vi "_PC_RTLoop_RTSysResource.vi"(7 "Function":enum16{"Init", "Get Data", "Close"}(ring)=enum."Get Data", 8 "error in (no error)":errorcluster, 11 "RT Resource XY Graph":refnum<vi>) -> (0 "error out":errorcluster)   [LabVIEW 2018]
uses:
  <resource>/objmgr/ni.var.rc
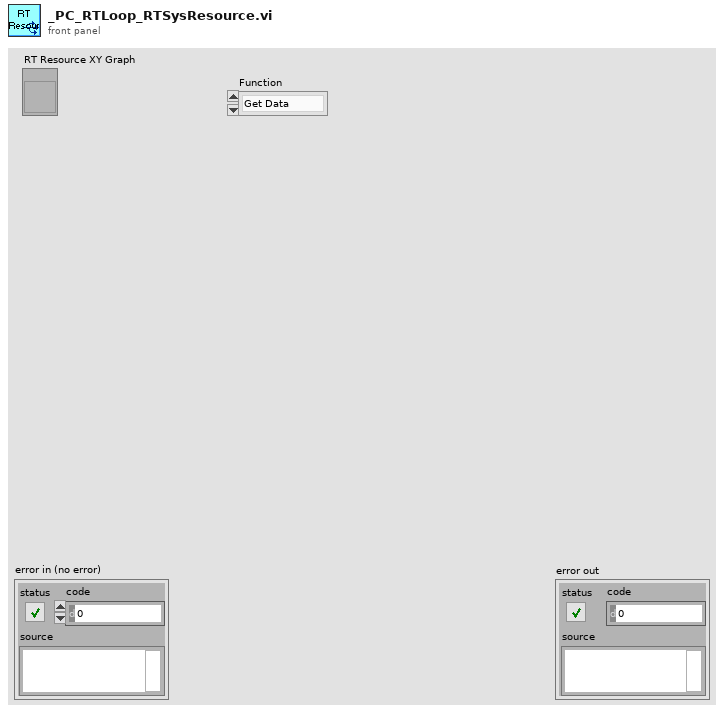
[diagram p1: front panel]
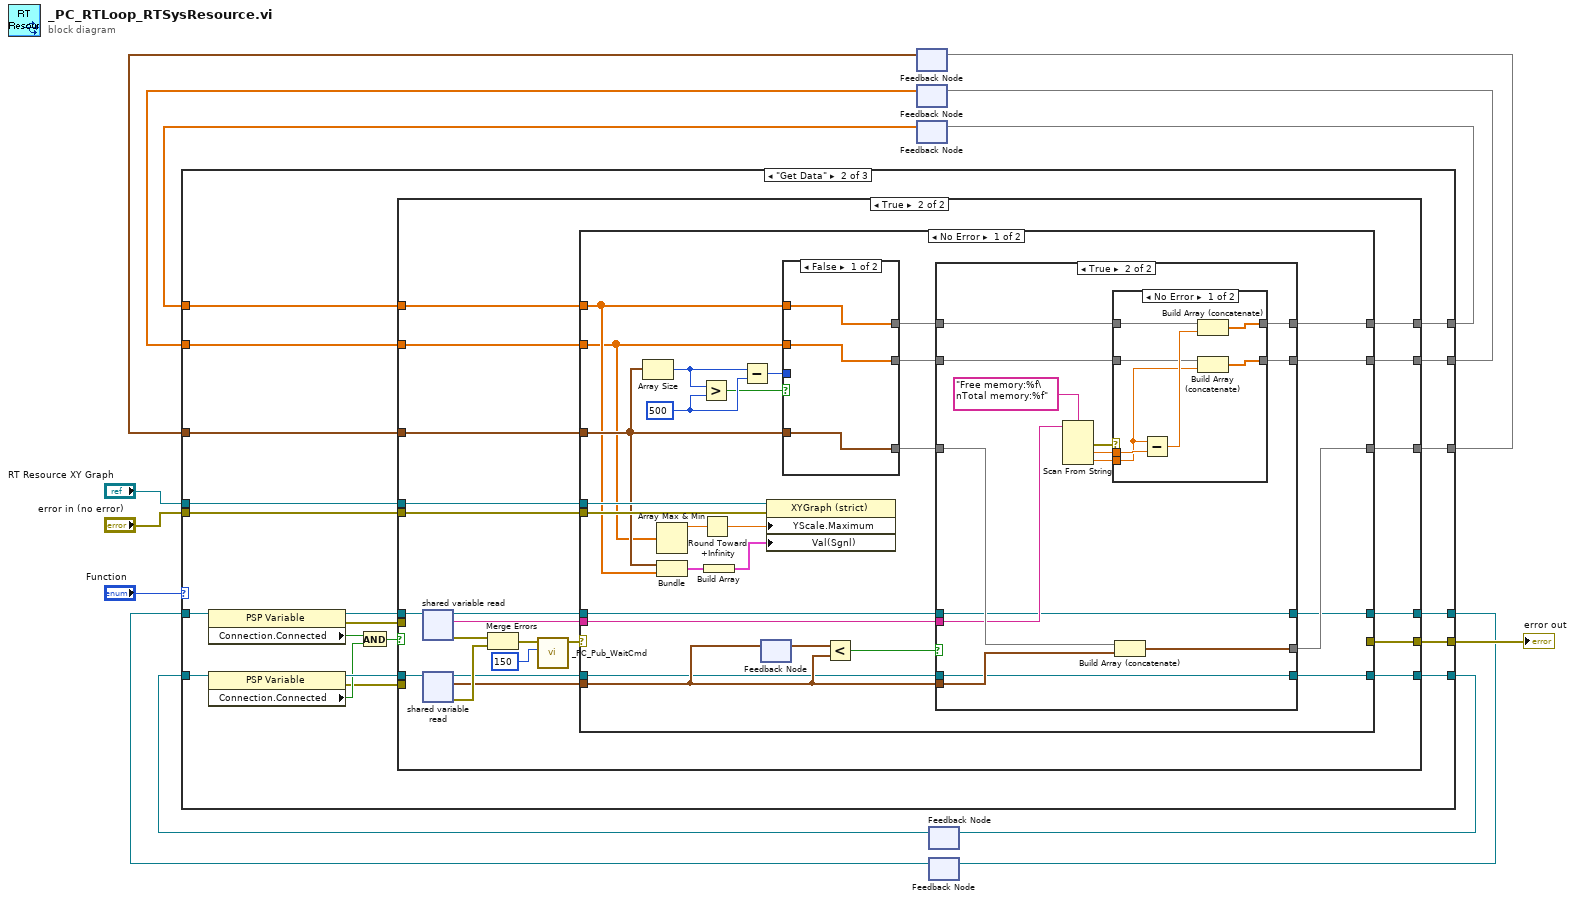
[diagram p0: block diagram]
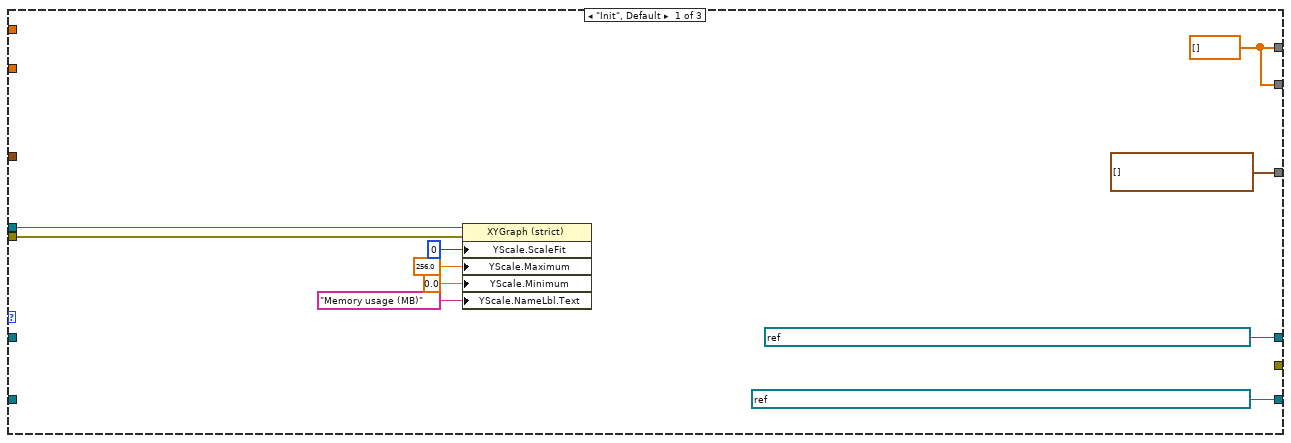
[diagram p2: hidden frame]
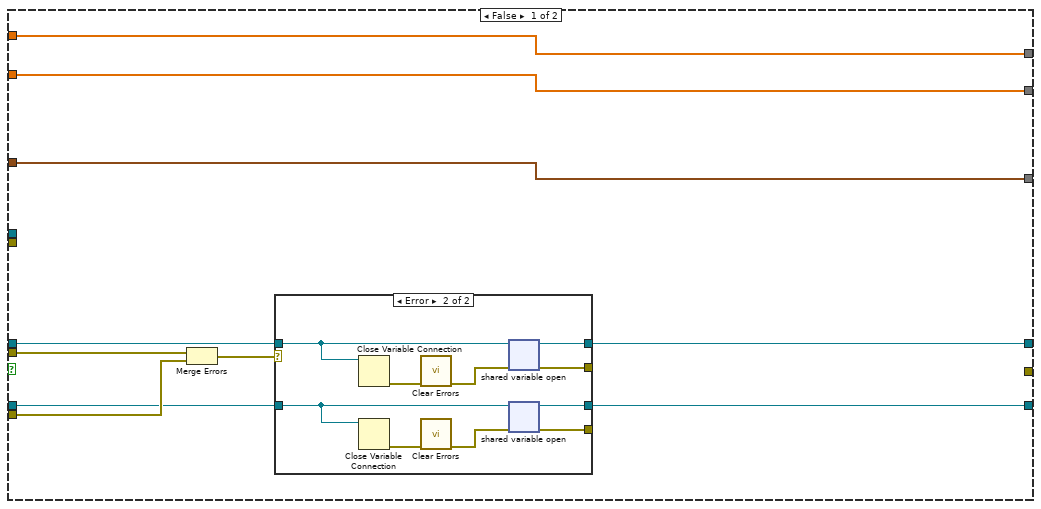
[diagram p3: hidden frame]
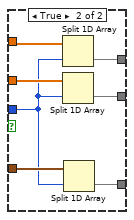
[diagram p7: hidden frame]
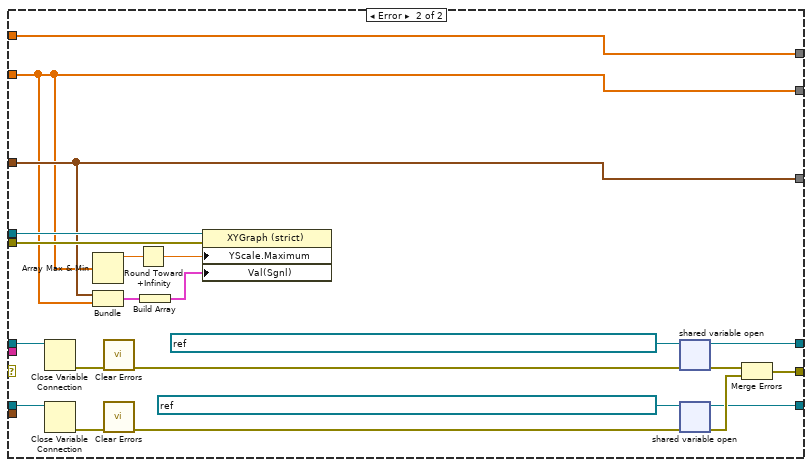
[diagram p8: hidden frame]
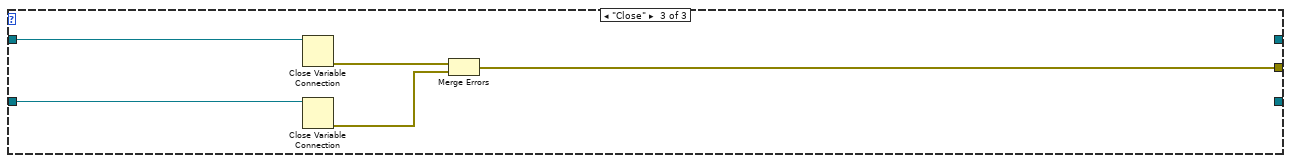
[diagram p9: hidden frame]
diagram:
  n1 = feedback #1() -> (w9:timestamp[])  [unwired: 1 in]
  n2 = feedback #2() -> (w11:dbl[])  [unwired: 1 in]
  n3 = feedback #3() -> (w13:dbl[])  [unwired: 1 in]
  n4 = feedback #4() -> (w5:refnum<k21>)  [unwired: 1 in]
  n5 = feedback #5() -> (w4:refnum<k21>)  [unwired: 1 in]
  n6 = case shown="\"Get Data\"" "Function" {
    tunnel: [w22 w44 _] -> w14
    tunnel: w13 -> [_ w43 _]
    tunnel: [w22 w42 _] -> w12
    tunnel: w11 -> [_ w41 _]
    tunnel: [timestamp[] [] w40 _] -> w10
    tunnel: w9 -> [_ w39 _]
    tunnel: [_ w38 w176] -> w8
    tunnel: [refnum<k21> "ni.var.psp://NI-sbRIO/_RT_CtrlLoop_ResourcesMonitor_Variables/RT_SysTimeStamp" ("shared variable refnum in") w37 _] -> w7
    tunnel: [refnum<k21> "ni.var.psp://NI-sbRIO/_RT_CtrlLoop_ResourcesMonitor_Variables/ResourceUsage" ("shared variable refnum in") w36 _] -> w6
    tunnel: w4 -> [_ w35 w180]
    tunnel: w5 -> [_ w34 w179]
    tunnel: "RT Resource XY Graph" -> [w16 w33 _]
    tunnel: "error in (no error)" -> [w15 w32 _]
    frame "Init", Default {
      w22 = dbl[] []
      n7 = property class="XYGraph (strict)"(reference=w16, error in=w15, "YScale.ScaleFit"=u8 0 ("Y Scale.Scale Fit"), "YScale.Maximum"=256.0 ("X Scale.Range:Maximum"), "YScale.Minimum"=0.0 ("X Scale.Range:Minimum"), "YScale.NameLbl.Text"="Memory usage (MB)" ("Y Scale.Name Label.Text")) -> ()  [unwired: 2 out]
    }
    frame "Get Data" {
      n8 = property class="PSP Variable"(reference=w35) -> (reference out=w31:refnum<k21>, error out=w26:errorcluster, "Connection.Connected"=w29:bool)  [unwired: 1 in]
      n9 = property class="PSP Variable"(reference=w34) -> (reference out=w30:refnum<k21>, error out=w25:errorcluster, "Connection.Connected"=w28:bool)  [unwired: 1 in]
      n10 = And(x=w29, y=w28) -> (x .and. y?=w27:bool)
      n11 = case shown="True" w27 {
        tunnel: [w54 w82] -> w44
        tunnel: w43 -> [w54 w81]
        tunnel: [w53 w80] -> w42
        tunnel: w41 -> [w53 w79]
        tunnel: [w52 w78] -> w40
        tunnel: w39 -> [w52 w77]
        tunnel: [_ w76] -> w38
        tunnel: [w46 w75] -> w37
        tunnel: [w45 w74] -> w36
        tunnel: w33 -> [_ w73]
        tunnel: w32 -> [_ w72]
        tunnel: w31 -> [w48 w68]
        tunnel: w30 -> [w47 w67]
        tunnel: w26 -> [w51 _]
        tunnel: w25 -> [w50 _]
        frame False {
          n12 = Merge Errors(w51, w50) -> (w49:errorcluster)
          n13 = case shown="Error" w49 {
            tunnel: w48 -> [w56 w64]
            tunnel: w47 -> [w55 w62]
            tunnel: [_ w60] -> _
            tunnel: [_ w59] -> _
            tunnel: [w55 w58] -> w46
            tunnel: [w56 w57] -> w45
            frame No Error {
            }
            frame Error {
              n14 = Close Variable Connection(11:w64) -> (0:w66:errorcluster)  [unwired: 1 in]
              n15 = Close Variable Connection(11:w62) -> (0:w65:errorcluster)  [unwired: 1 in]
              n16 = call <vilib>:"Clear Errors.vi"("error in (no error)"=w66) -> ("error out"=w63:errorcluster)  [unwired: 5 in, 1 out]
              n17 = call <vilib>:"Clear Errors.vi"("error in (no error)"=w65) -> ("error out"=w61:errorcluster)  [unwired: 5 in, 1 out]
              n18 = shared-variable-open(w64, w63) -> (w57:refnum<k21>, w60:errorcluster)
              n19 = shared-variable-open(w62, w61) -> (w58:refnum<k21>, w59:errorcluster)
            }
          }
        }
        frame True {
          n20 = shared-variable-read(w68) -> (w86:refnum<k21>, w88:errorcluster, w85:string)  [unwired: 1 in]
          n21 = shared-variable-read(w67) -> (w84:refnum<k21>, w87:errorcluster, w83:timestamp)  [unwired: 1 in]
          n22 = Merge Errors(w88, w87) -> (w71:errorcluster)
          n23 = call "_PC_Pub_WaitCmd.vi"("milliseconds to wait"=u32 150, "error in (no error)"=w71) -> ("error out"=w70:errorcluster)  [unwired: 9 in]
          n24 = case shown="No Error" w70 {
            tunnel: w86 -> [w92 w162]
            tunnel: w85 -> [w108 _]
            tunnel: w84 -> [w90 w161]
            tunnel: w83 -> [w105 _]
            tunnel: [w95 w175] -> w82
            tunnel: w81 -> [w97 w175]
            tunnel: w79 -> [w96 w167]
            tunnel: [w94 w167] -> w80
            tunnel: w77 -> [w98 w168]
            tunnel: [w93 w168] -> w78
            tunnel: w73 -> [w100 w170]
            tunnel: w72 -> [w99 w169]
            tunnel: [_ w156] -> w76
            tunnel: [w91 w155] -> w74
            tunnel: [w89 w154] -> w75
            frame No Error {
              w114 = 500 ("y")
              n25 = Array Size(array=w98) -> (size(s)=w115:i32)
              n26 = Array Max & Min(array=w96) -> (max value=w102:dbl)  [unwired: 3 out]
              n27 = Bundle(w98, w97) -> (w104:cluster{timestamp[], dbl[]})  [unwired: 1 in]
              n28 = Greater?(x=w115, y=w114) -> (0:w113:bool)
              n29 = Round Toward +Infinity(x=w102) -> (ceil(x): smallest int >= x=w101:dbl)
              n30 = Build Array(w104) -> (w103:cluster{timestamp[], dbl[]}[])
              n31 = Subtract(x=w115, y=w114) -> (x-y=w112:i32)
              n32 = feedback #6() -> (w106:timestamp)  [unwired: 1 in]
              n33 = feedback-in #6(w105) -> ()
              n34 = property class="XYGraph (strict)"(reference=w100, error in=w99, "YScale.Maximum"=w101, "Val(Sgnl)"=w103) -> ()  [unwired: 2 out]
              n35 = case shown="False" w113 {
                tunnel: w112 -> [_ w148]
                tunnel: w98 -> [w144 w153]
                tunnel: [w144 w152] -> w109
                tunnel: w96 -> [w145 w151]
                tunnel: [w145 w150] -> w110
                tunnel: w97 -> [w146 w149]
                tunnel: [w146 w147] -> w111
                frame False {
                }
                frame True {
                  n36 = Split 1D Array(array=w149, index=w148) -> (second subarray=w147:dbl[])  [unwired: 1 out]
                  n37 = Split 1D Array(array=w151, index=w148) -> (second subarray=w150:dbl[])  [unwired: 1 out]
                  n38 = Split 1D Array(array=w153, index=w148) -> (second subarray=w152:timestamp[])  [unwired: 1 out]
                }
              }
              n39 = Less?(x=w106, y=w105) -> (x < y?=w107:bool)
              n40 = case shown="True" w107 {
                tunnel: [w120 w134] -> w95
                tunnel: [w119 w129] -> w94
                tunnel: [w118 w133] -> w93
                tunnel: w109 -> [w118 w132]
                tunnel: w111 -> [w120 w131]
                tunnel: w110 -> [w119 w128]
                tunnel: w105 -> [_ w130]
                tunnel: w108 -> [_ w127]
                tunnel: w92 -> [w117 w122]
                tunnel: [w117 w122] -> w91
                tunnel: w90 -> [w116 w121]
                tunnel: [w116 w121] -> w89
                frame False {
                }
                frame True {
                  n41 = Scan From String(format string="Free memory:%f\nTotal memory:%f", input string=w127) -> (error out=w123:errorcluster, output 1=w125:dbl, output 2=w124:dbl)  [unwired: 4 in, 2 out]
                  n42 = case shown="No Error" w123 {
                    tunnel: [w141 w143] -> w134
                    tunnel: w131 -> [w140 w143]
                    tunnel: [w139 w142] -> w129
                    tunnel: w128 -> [w137 w142]
                    tunnel: w125 -> [w136 _]
                    tunnel: w124 -> [w135 _]
                    frame No Error {
                      n43 = Subtract(x=w135, y=w136) -> (x-y=w138:dbl)
                      n44 = Build Array (concatenate)(w140, w138) -> (w141:dbl[])
                      n45 = Build Array (concatenate)(w137, w135) -> (w139:dbl[])
                    }
                    frame Error {
                    }
                  }
                  n46 = Build Array (concatenate)(w132, w130) -> (w133:timestamp[])
                }
              }
            }
            frame Error {
              n47 = Close Variable Connection(11:w162) -> (0:w166:errorcluster)  [unwired: 1 in]
              n48 = Close Variable Connection(11:w161) -> (0:w165:errorcluster)  [unwired: 1 in]
              n49 = Array Max & Min(array=w167) -> (max value=w172:dbl)  [unwired: 3 out]
              n50 = Bundle(w168, w167) -> (w174:cluster{timestamp[], dbl[]})  [unwired: 1 in]
              n51 = call <vilib>:"Clear Errors.vi"("error in (no error)"=w166) -> ("error out"=w164:errorcluster)  [unwired: 5 in, 1 out]
              n52 = call <vilib>:"Clear Errors.vi"("error in (no error)"=w165) -> ("error out"=w163:errorcluster)  [unwired: 5 in, 1 out]
              n53 = Round Toward +Infinity(x=w172) -> (ceil(x): smallest int >= x=w171:dbl)
              n54 = Build Array(w174) -> (w173:cluster{timestamp[], dbl[]}[])
              n55 = property class="XYGraph (strict)"(reference=w170, error in=w169, "YScale.Maximum"=w171, "Val(Sgnl)"=w173) -> ()  [unwired: 2 out]
              n56 = shared-variable-open(refnum<k21> "ni.var.psp://NI-sbRIO/_RT_CtrlLoop_ResourcesMonitor_Variables/ResourceUsage" ("shared variable refnum in"), w164) -> (w155:refnum<k21>, w158:errorcluster)
              n57 = shared-variable-open(refnum<k21> "ni.var.psp://NI-sbRIO/_RT_CtrlLoop_ResourcesMonitor_Variables/RT_SysTimeStamp" ("shared variable refnum in"), w163) -> (w154:refnum<k21>, w157:errorcluster)
              n58 = Merge Errors(w158, w157) -> (w156:errorcluster)
            }
          }
        }
      }
    }
    frame "Close" {
      n59 = Close Variable Connection(11:w180) -> (0:w178:errorcluster)  [unwired: 1 in]
      n60 = Close Variable Connection(11:w179) -> (0:w177:errorcluster)  [unwired: 1 in]
      n61 = Merge Errors(w178, w177) -> (w176:errorcluster)
    }
  }
  "error out" <- w8
  n62 = feedback-in #1(w10) -> ()
  n63 = feedback-in #2(w12) -> ()
  n64 = feedback-in #3(w14) -> ()
  n65 = feedback-in #4(w7) -> ()
  n66 = feedback-in #5(w6) -> ()
